vi "全局-模拟器变量.vi"() -> ()   [LabVIEW 2017]
panel:
  out "vi引用[]":refnum<vi>[](array[refnum])
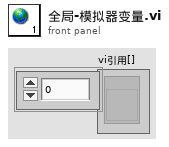
[diagram p1: front panel]
diagram:
